vi "ReadModbus.vi"(8 "error in (no error)":errorcluster, 11 "Modbus master in":refnum<class "Modbus Master.lvclass">) -> (0 "error out":errorcluster)   [LabVIEW 2018, in "Modbus.lvlib"]
uses:
  Modbus.lvlib
  <vilib>/Modbus/master/Modbus Master.lvclass
  <userlib>/_OpenG.lib/array/array.llb/Reorder 1D Array2 (DBL)__ogtk.vi
  RT-UDP Writer/UDP Writer.lvlib
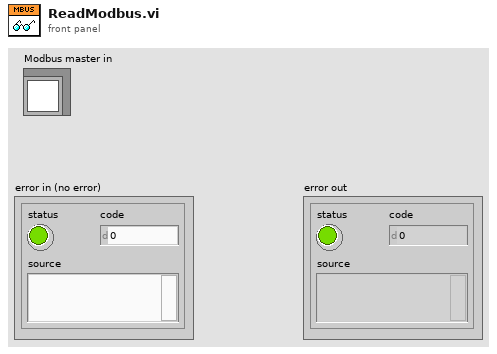
[diagram p1: front panel]
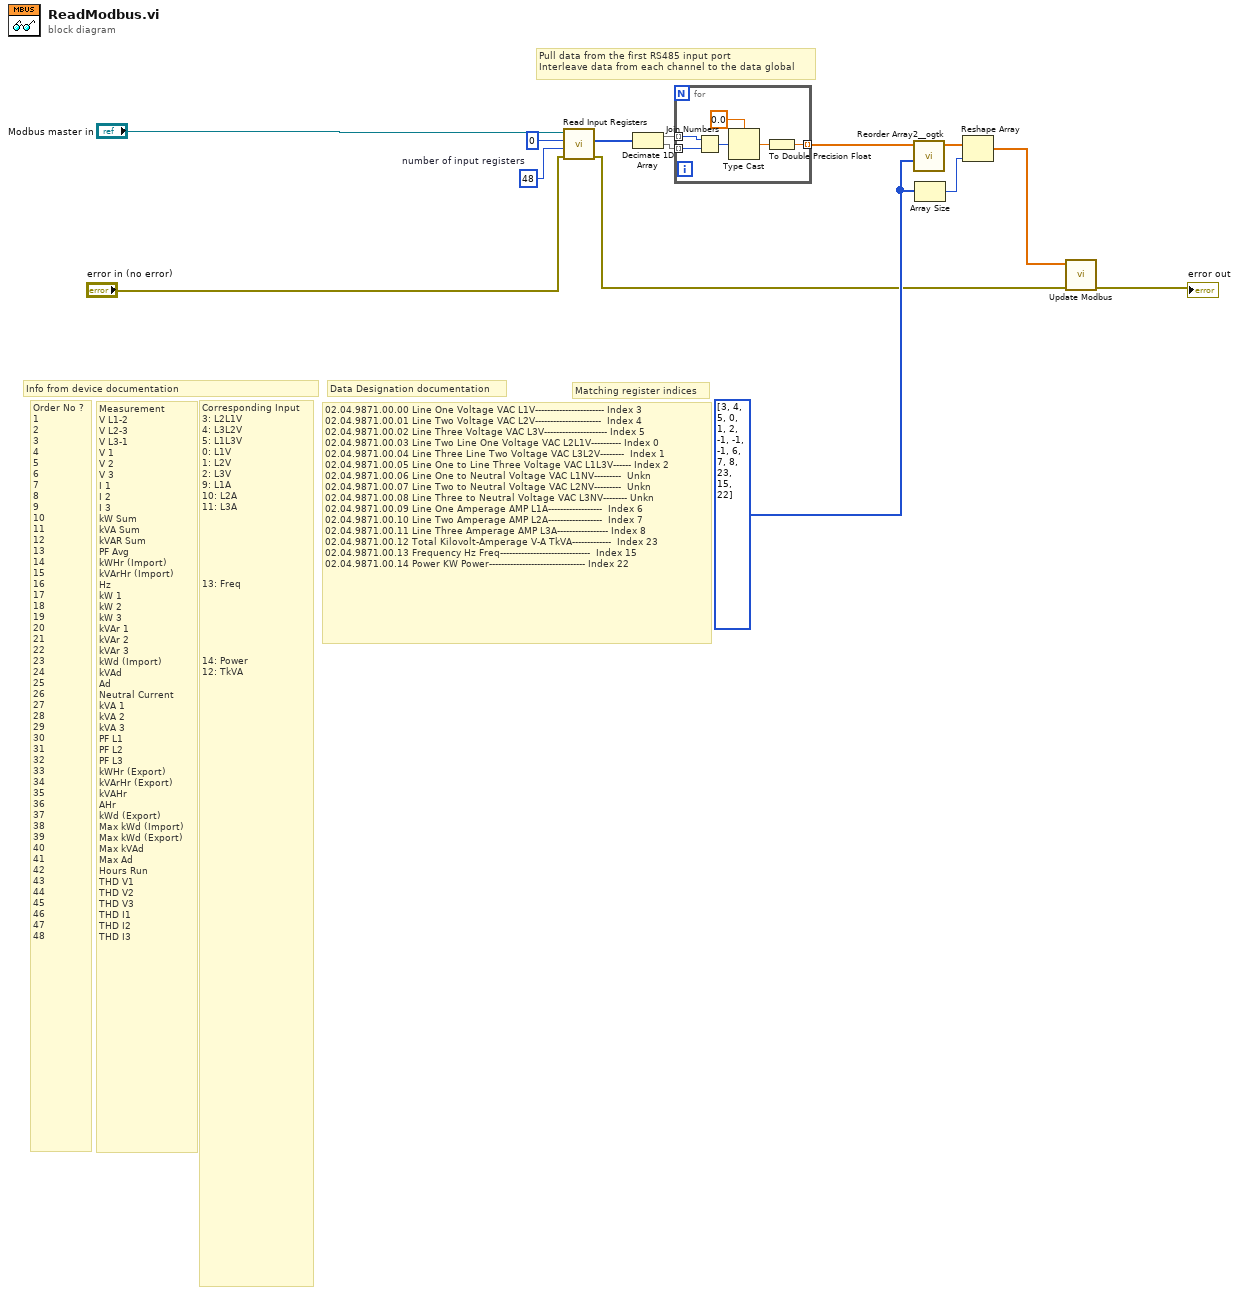
[diagram p0: block diagram]
diagram:
  w6 = u16 48  # number of input registers
  w12 = i32[] [3, 4, 5, 0, 1, 2, -1, -1, -1, 6, 7, 8, 23, 15, 22] ("indices")
  # "Matching register indices"
  # "Data Designation documentation"
  # "Info from device documentation"
  # "Corresponding Input\n3: L2L1V\n4: L3L2V\n5: L1L3V\n0: L1V\n1: L2V\n2: L3V\n9: L1A\n10: L2A\n11: L3A\n\n\n\n\n\n\n13: Freq\n\n\n\n\n\n\n14: Power\n12: TkVA"
  # "Order No\t?\n1\t\n2\t\n3\t\n4\t\n5\t\n6\t\n7\t\n8\t\n9\t\n10\t\n11\t\n12\t\n13\t\n14\t\n15\t\n16\t\n17\t\n18\t\n19\t\n20\t\n21\t\n22\t\n23\t\n24\t\n25\t\n26\t\n27\t\n28\t\n29\t\n30\t\n31\t\n32\t\n33\t\n34\t\n35\t\n36\t\n37\t\n38\t\n39\t\n40\t\n41\t\n42\t\n43\t\n44\t\n45\t\n46\t\n47\t\n48"
  # "Measurement\nV L1-2\nV L2-3\nV L3-1\nV 1\nV 2\nV 3\nI 1\nI 2\nI 3\nkW Sum\nkVA Sum\nkVAR Sum\nPF Avg\nkWHr (Import)\nkVArHr (Import)\nHz\nkW 1\nkW 2\nkW 3\nkVAr 1\nkVAr 2\nkVAr 3\nkWd (Import)\nkVAd\nAd\nNeutral Current\nkVA 1\nkVA 2\nkVA 3\nPF L1\nPF L2\nPF L3\nkWHr (Export)\nkVArHr (Export)\nkVAHr\nAHr\nkWd (Export)\nMax kWd (Import)\nMax kWd (Export)\nMax kVAd\nMax Ad\nHours Run\nTHD V1\nTHD V2\nTHD V3\nTHD I1\nTHD I2\nTHD I3"
  # "02.04.9871.00.00\tLine One Voltage\tVAC\tL1V----------------------- Index 3\n02.04.9871.00.01\tLine Two Voltage\tVAC\tL2V----------------------  Index 4\n02.04.9871.00.02\tLine Three Voltage\tVAC\tL3V--------------------- Index 5\n02.04.9871.00.03\tLine Two Line One Voltage\tVAC\tL2L1V---------- Index 0\n02.04.9871.00.04\tLine Three Line Two Voltage\tVAC\tL3L2V--------  Index 1\n02.04.9871.00.05\tLine One to Line Three Voltage\tVAC\tL1L3V------ Index 2\n02.04.9871.00.06\tLine One to Neutral Voltage\tVAC\tL1NV---------  Unkn\n02.04.9871.00.07\tLine Two to Neutral Voltage\tVAC\tL2NV---------  Unkn\n02.04.9871.00.08\tLine Three to Neutral Voltage\tVAC\tL3NV-------- Unkn\n02.04.9871.00.09\tLine One Amperage\tAMP\tL1A------------------  Index 6\n02.04.9871.00.10\tLine Two Amperage\tAMP\tL2A------------------  Index 7\n02.04.9871.00.11\tLine Three Amperage\tAMP\tL3A----------------- Index 8\n02.04.9871.00.12\tTotal Kilovolt-Amperage\tV-A\tTkVA-------------  Index 23\n02.04.9871.00.13\tFrequency\tHz\tFreq------------------------------  Index 15\n02.04.9871.00.14\tPower\tKW\tPower-------------------------------- Index 22"
  # "Pull data from the first RS485 input port\nInterleave data from each channel to the data global"
  n1 = call-dynamic "Read Input Registers.vi"("error in (no error)"="error in (no error)", "number of input registers"=w6, "starting address"=0 ("Starting index"), "Modbus master in"="Modbus master in") -> ("error out"=w3:errorcluster, "register values"=w10:u16[])  [unwired: 5 in, 1 out]
  n2 = Decimate 1D Array(w10) -> (w8:u16[], w9:u16[])
  n3 = for {
    tunnel: w8 -> [w19] mode=indexing
    tunnel: w9 -> [w18] mode=indexing
    tunnel: [w15] -> w13 mode=indexing
    n4 = Join Numbers(hi=w19, lo=w18) -> ((hi.lo)=w17:u32)
    n5 = Type Cast(type=sgl 0.0, x=w17) -> (*(type *) &x=w16:sgl)
    n6 = To Double Precision Float(number=w16) -> (double precision float=w15:dbl)
  }
  n7 = call-poly <userlib>:"Reorder Array2__ogtk.vi"("indices"=w12, "array"=w13) -> ("reordered array"=w14:dbl[])  [unwired: 9 in]
  n8 = Array Size(array=w12) -> (size(s)=w11:i32)
  n9 = Reshape Array(w14, w11) -> (w1:dbl[])
  n10 = call "Update Modbus.vi"("error in"=w3, "Modbus"=w1) -> ("error out"=→"error out":errorcluster)  [unwired: 9 in]
